vi "UI trackingXY CUDA.vi"(10 "ROI descriptors":T2[](array[typedef]) {"Contours"."Type" items=["No Selection", "Point", "Line", "Rectangle", "Oval", "Polygon", "Freehand Region", "Annulus", "Unused2", "Unused3", "Broken Line", "Freehand Line", "Rotated Rectangle"]}, 11 "image ref":T3[](array[typedef])) -> (2 "tracking out":T1[](array[typedef]) {"centroid"."Y Centroid" format="%.2f"; "centroid"."X Centroid" format="%.2f"; "ROI Des out"."Contours"."Type" items=["No Selection", "Point", "Line", "Rectangle", "Oval", "Polygon", "Freehand Region", "Annulus", "Unused2", "Unused3", "Broken Line", "Freehand Line", "Rotated Rectangle"]}, 3 "rdp_mean":dbl[][](array[numeric]))   [LabVIEW 2017]
uses:
  <vilib>/vision/Image Controls.llb/IMAQ Image.ctl
  control/Bead track.ctl
panel:
  in  "Centroid":cluster{"X Centroid":sgl, "Y Centroid":sgl} {"Y Centroid" format="%.2f"; "X Centroid" format="%.2f"}
  out "x_qi_out":sgl[][](array[numeric])
  out "y_qi_out":sgl[][](array[numeric])
  out "rdp_profile":sgl[][][](array[numeric])
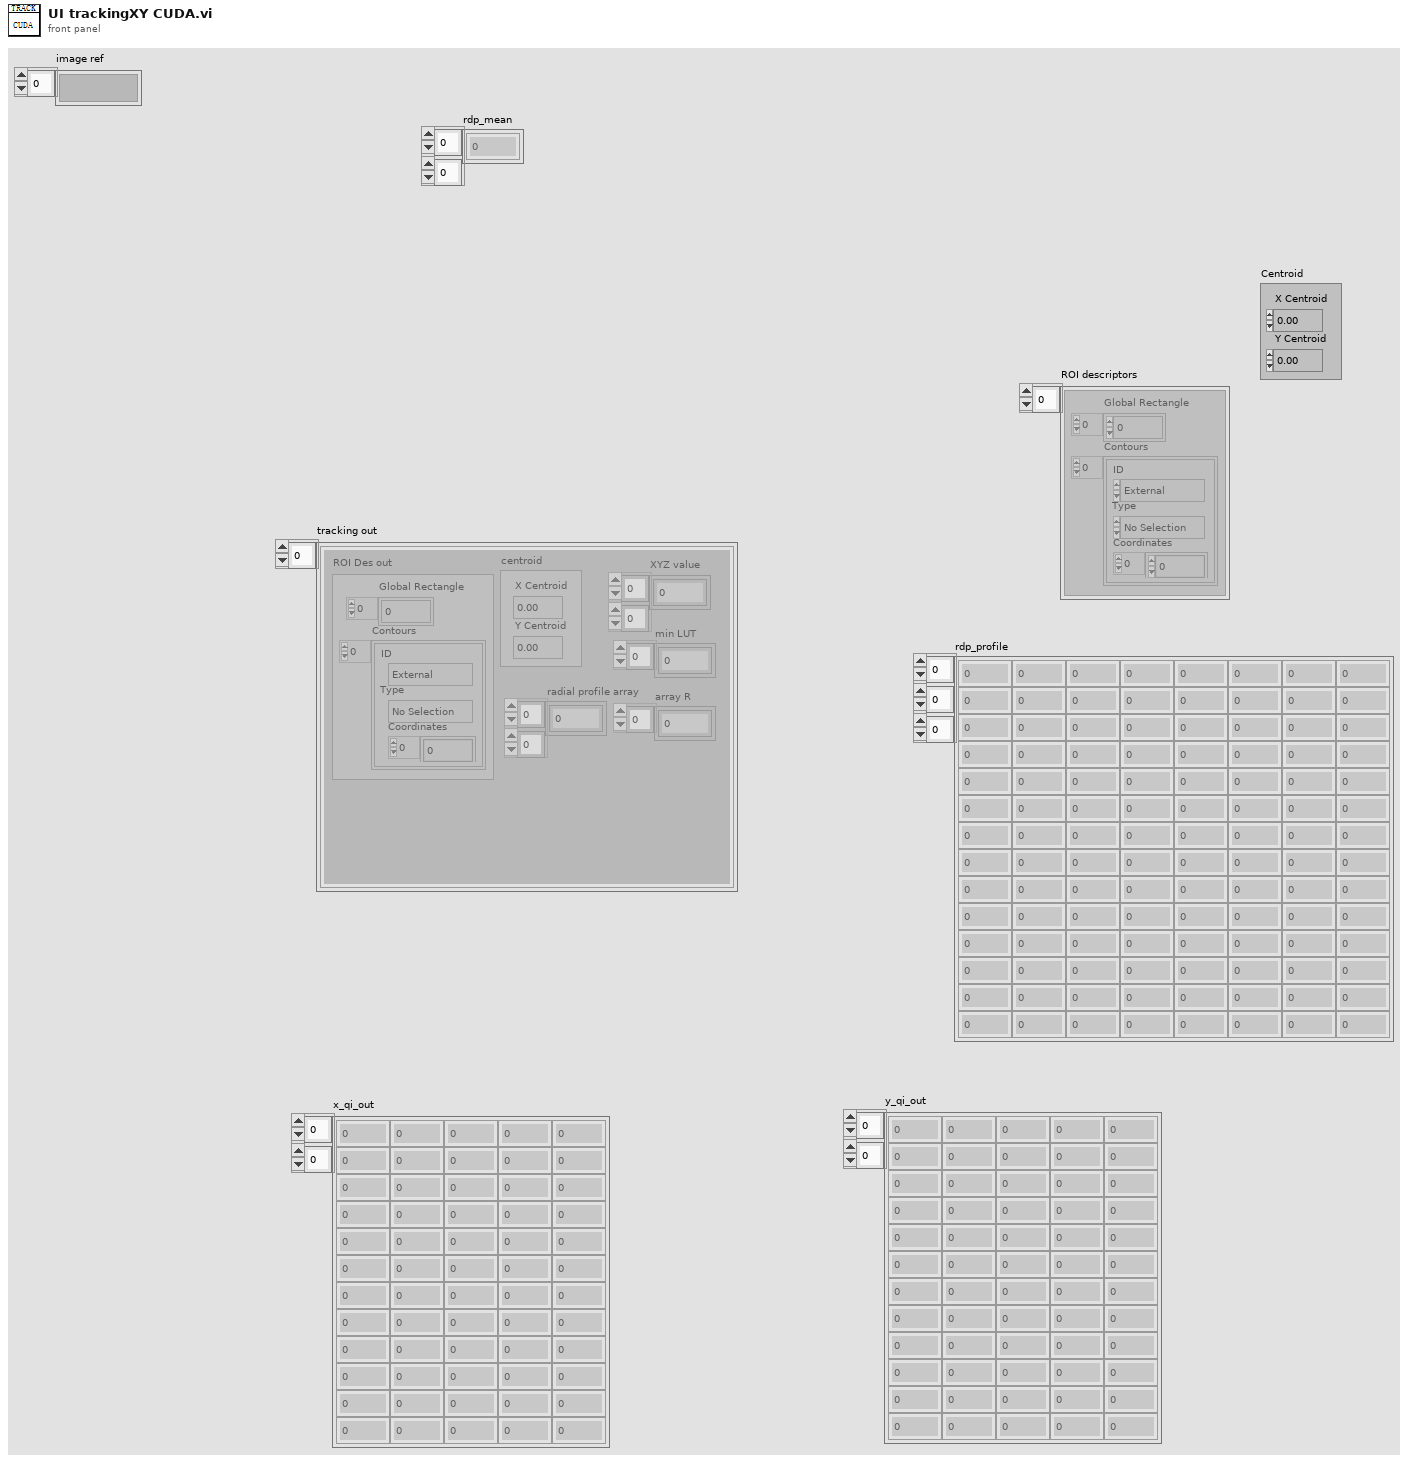
[diagram p1: front panel]
types:
  T1 = typedef "Bead track.ctl" = cluster{"XYZ value":dbl[][], "radial profile array":dbl[][], "min LUT":dbl[], "ROI Des out":T2, "array R":dbl[], "centroid":cluster{"X Centroid":sgl, "Y Centroid":sgl}}
  T2 = typedef "ROI Descriptor" = cluster{"Global Rectangle":i32[], "Contours":cluster{"ID":enum32{"External", "Internal"}, "Type":u32, "Coordinates":i32[]}[]}
  T3 = typedef "IMAQ Image.ctl" = refnum<image>
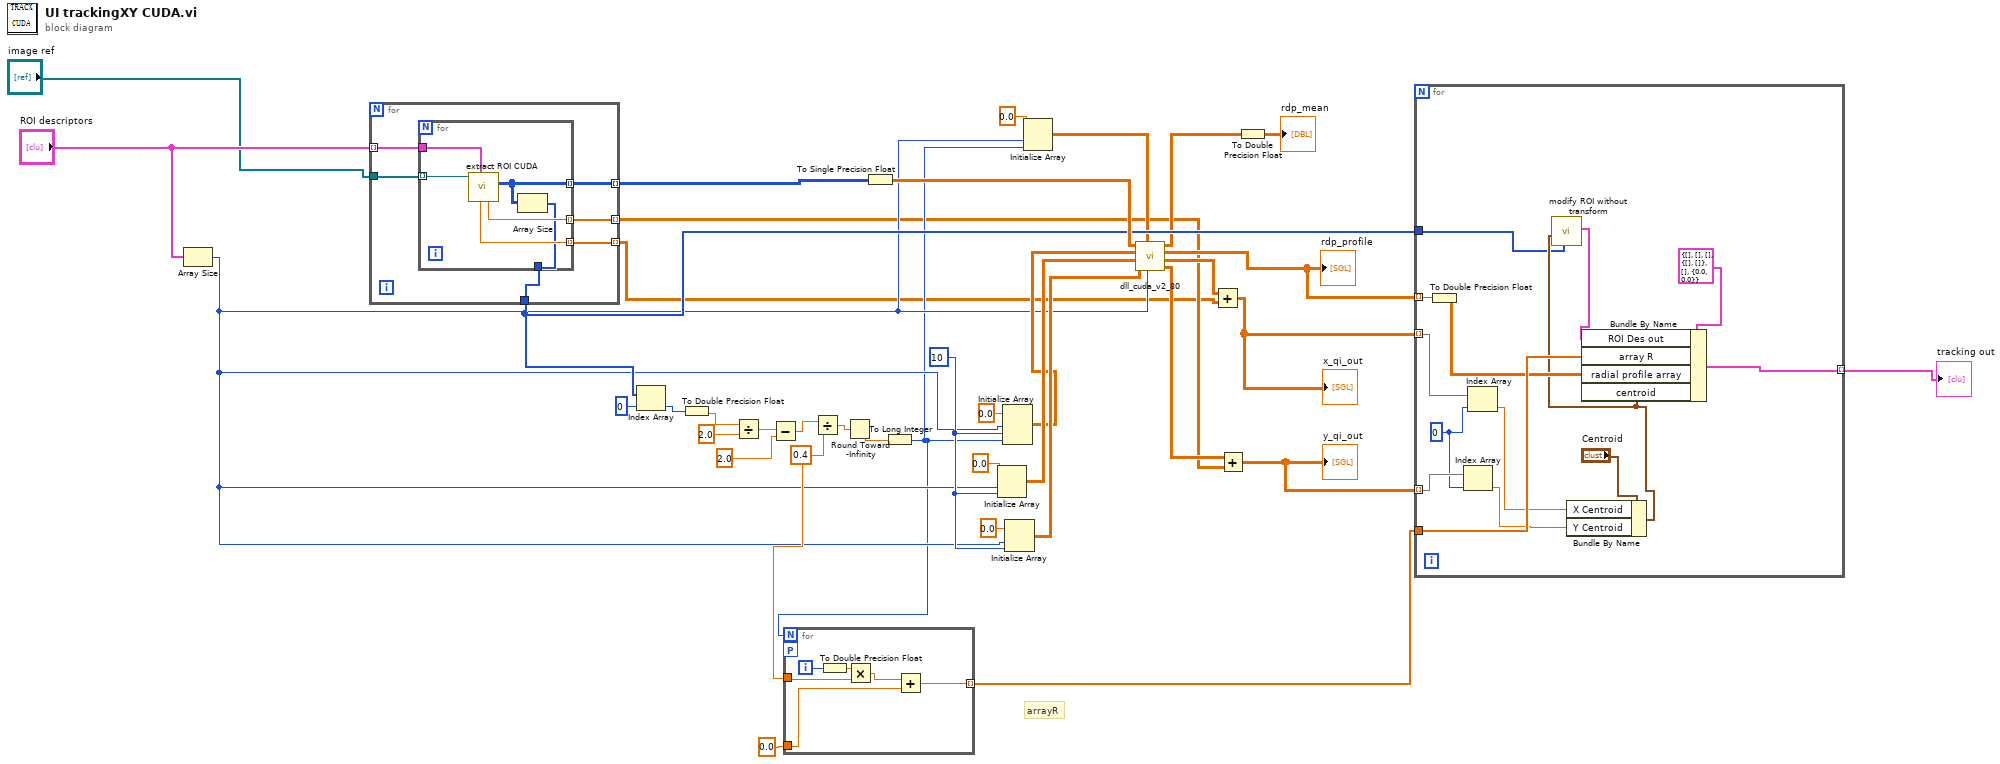
[diagram p0: block diagram]
diagram:
  w11 = 10 ("n_frame")
  w20 = 0.4 ("y")
  # "arrayR"
  n1 = Array Size(array="ROI descriptors") -> (size(s)=w9:i32)
  n2 = for {
    tunnel: "image ref" -> [w44]
    tunnel: "ROI descriptors" -> [w43] mode=indexing
    tunnel: [w42] -> w26 mode=indexing
    tunnel: [w41] -> w1 mode=indexing
    tunnel: [w40] -> w2 mode=indexing
    tunnel: [w39] -> w13
    n3 = for {
      tunnel: w44 -> [w50] mode=indexing
      tunnel: w43 -> [w49]
      tunnel: [w45] -> w42 mode=indexing
      tunnel: [w48] -> w41 mode=indexing
      tunnel: [w47] -> w40 mode=indexing
      tunnel: [w46] -> w39
      n4 = call "extract ROI CUDA.vi"("ROI Descriptor"=w49, "CCD image ref"=w50) -> ("ROI array out"=w45:u8[][], "Y_base"=w47:sgl, "X_base"=w48:sgl)  [unwired: 7 in]
      n5 = Array Size(array=w45) -> (size(s)=w46:i32[])
    }
  }
  n6 = Index Array(array=w13, index=0) -> (element=w6:i32)
  n7 = To Double Precision Float(number=w6) -> (double precision float=w38:dbl)
  n8 = Divide(x=w38, y=2.0) -> (x/y=w37:dbl)
  n9 = Subtract(x=w37, y=2.0) -> (x-y=w36:dbl)
  n10 = Divide(x=w36, y=w20) -> (x/y=w35:dbl)
  n11 = Round Toward -Infinity(1:w35) -> (0:w34:dbl)
  n12 = To Single Precision Float(number=w26) -> (single precision float=w25:sgl[][][][])
  n13 = To Long Integer(number=w34) -> (32bit integer=w8:i32)
  n14 = for "For循环" {
    N: w8 -> [_]
    tunnel: 0.0 ("R_min") -> [w53]
    tunnel: w20 -> [w55]
    tunnel: [w51] -> w16 mode=indexing
    workers-P: _ -> [_]
    i -> [w56]
    n15 = To Double Precision Float(number=w56) -> (double precision float=w52:dbl)
    n16 = Multiply(x=w52, y=w55) -> (x*y=w54:dbl)
    n17 = Add(x=w54, y=w53) -> (x+y=w51:dbl)
  }
  n18 = Initialize Array(sgl 0.0 ("element"), w9, w11) -> (w24:sgl[][])
  n19 = Initialize Array(sgl 0.0 ("element"), w9, w11, w8) -> (w23:sgl[][][])
  n20 = Initialize Array(sgl 0.0 ("element"), w9, w11) -> (w28:sgl[][])
  n21 = Initialize Array(sgl 0.0 ("element"), w9, w8) -> (w7:sgl[][])
  n22 = call "dll_cuda_v2_80.vi"("n_stream"=w9, "rdp_mean"=w7, "yc"=w28, "xc"=w24, "rdp_profile"=w23, "img_mat 4d"=w25) -> ("yc out"=w22:sgl[][], "xc out"=w14:sgl[][], "rdp_profile out"=w19:sgl[][][], "rdp_mean out"=w4:sgl[][])  [unwired: 2 in]
  "rdp_profile" <- w19
  n23 = Add(x=w14, y=w1) -> (x+y=w18:sgl[][])
  "x_qi_out" <- w18
  n24 = Add(x=w22, y=w2) -> (x+y=w17:sgl[][])
  "y_qi_out" <- w17
  n25 = To Double Precision Float(number=w4) -> (double precision float=→"rdp_mean":dbl[][])
  n26 = for {
    tunnel: w19 -> [w68] mode=indexing
    tunnel: w18 -> [w66] mode=indexing
    tunnel: w17 -> [w65] mode=indexing
    tunnel: w16 -> [w69]
    tunnel: w13 -> [w59]
    tunnel: [w57] -> w5 mode=indexing
    w64 = 0
    n27 = To Double Precision Float(number=w68) -> (double precision float=w67:dbl[][])
    n28 = Index Array(array=w65, index=w64) -> (element=w61:sgl)
    n29 = Index Array(array=w66, index=w64) -> (element=w62:sgl)
    n30 = Bundle By Name(cluster="Centroid", "X Centroid"=w62, "Y Centroid"=w61) -> (w60:cluster{"X Centroid":sgl, "Y Centroid":sgl})
    n31 = call "modify ROI without transform.vi"("ROI size num"=w59, "new x y"=w60) -> ("ROI Descriptor out"=w58:T2)  [unwired: 8 in, 1 out]
    n32 = Bundle By Name(cluster=T1 {"XYZ value"=[], "radial profile array"=[], "min LUT"=[], "ROI Des out"={"Global Rectangle"=[], "Contours"=[]}, "array R"=[], "centroid"={"X Centroid"=0.0, "Y Centroid"=0.0}} ("tracking"), "ROI Des out"=w58, "array R"=w69, "radial profile array"=w67, "centroid"=w60) -> (w57:T1)
  }
  "tracking out" <- w5
